vi "计算图像重排一维数组.vi"(1 "优化图像簇":T1) -> (0 "图像重排一维数组":dbl[](array[numeric]))   [LabVIEW 2018]
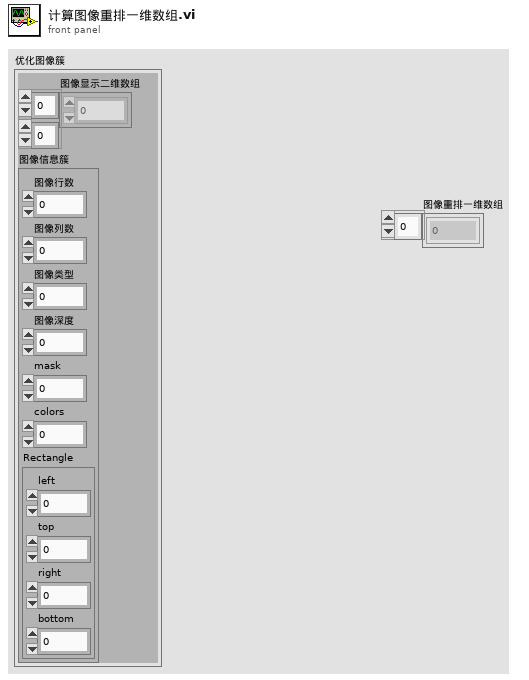
[diagram p1: front panel]
types:
  T1 = cluster{"图像显示二维数组":dbl[][], "图像信息簇":cluster{"图像行数":dbl, "图像列数":dbl, "图像类型":dbl, "图像深度":i32, "mask":i32, "colors":i32, "Rectangle":cluster{"left":i16, "top":i16, "right":i16, "bottom":i16}}}
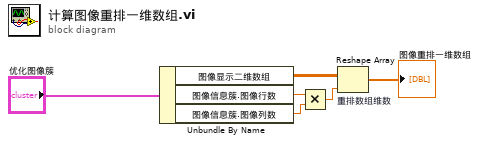
[diagram p0: block diagram]
diagram:
  n1 = Unbundle By Name("优化图像簇") -> ("图像显示二维数组"=w5:dbl[][], "图像信息簇.图像行数"=w4:dbl, "图像信息簇.图像列数"=w3:dbl)
  n2 = Multiply(x=w4, y=w3) -> (x*y=w2:dbl)
  n3 = Reshape Array "重排数组维数"(w5, w2) -> (→"图像重排一维数组":dbl[])
